vi "querySignalInterface.vi"(8 "error in (no error)":errorcluster, 11 "IBaseObject in":refnum<class "IBaseObject.lvclass">) -> (0 "error out":errorcluster, 2 "ISignal out":refnum<class "ISignal.lvclass">, 3 "IBaseObject out":refnum<class "IBaseObject.lvclass">)   [LabVIEW 2022 SP3, in "openDAQ.lvlib" / "IBaseObject.lvlib" / "IBaseObject.lvclass"]
uses:
  <instrlib>/openDAQ/Public/Classes/IBaseObject/IBaseObject.lvclass
  <instrlib>/openDAQ/Public/Classes/IBaseObject/IBaseObject.lvclass/IBaseObject.ctl
  <instrlib>/openDAQ/Binaries/Windows/x86/copendaq32.dll
  <instrlib>/openDAQ/Public/Classes/ISignal/ISignal.lvclass
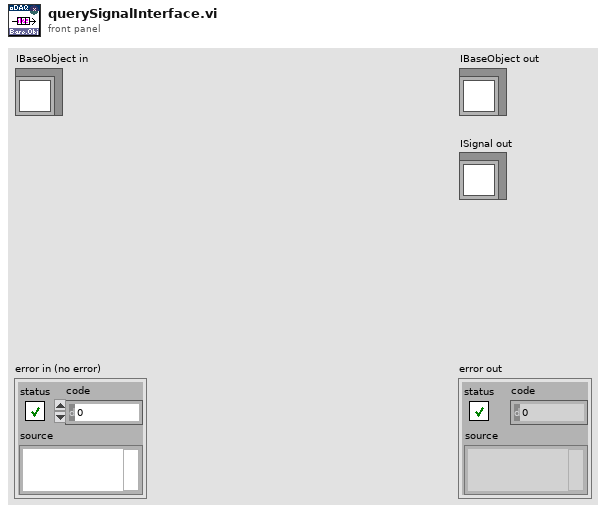
[diagram p1: front panel]
types:
  T1 = enum16{"big-endian, network order", "native, host order", "little-endian"}
  T2 = cluster{"status":bool, "code":u32, "source":string}
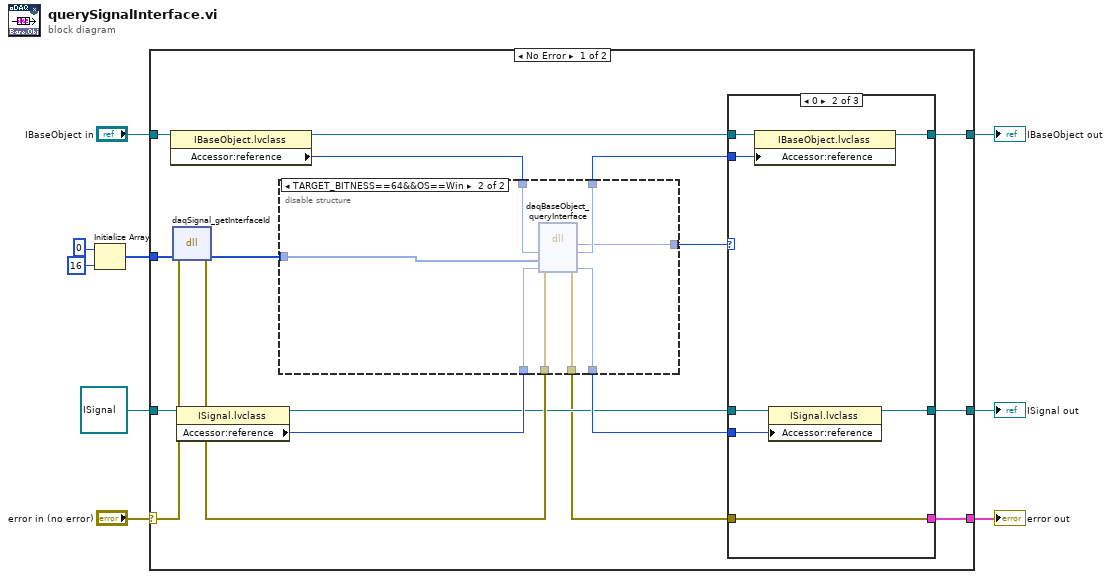
[diagram p0: block diagram]
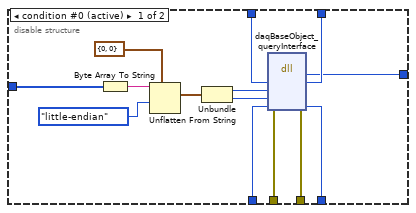
[diagram p2: hidden frame]
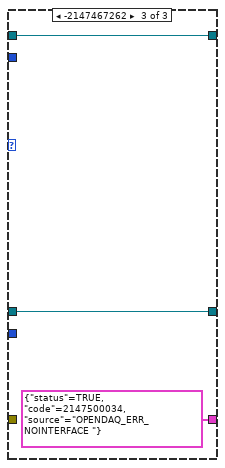
[diagram p4: hidden frame]
diagram:
  n1 = Initialize Array(u8 0, 16 ("dimension size")) -> (w1:u8[])
  n2 = case shown="No Error" "error in (no error)" {
    selector: "error in (no error)" -> [w22 w64]
    tunnel: [w12 w64] -> w8
    tunnel: [w19 w63] -> w6
    tunnel: "IBaseObject in" -> [w26 w63]
    tunnel: refnum<class "ISignal.lvclass"> refnum ("openDAQ.lvlib:IBaseObject.lvlib:IPropertyObject.lvlib:IComponent.lvlib:ISignal.lvlib:ISignal.lvclass") -> [w25 w62]
    tunnel: [w15 w62] -> w4
    tunnel: w1 -> [w11 _]
    frame No Error {
      n3 = property class="IBaseObject.lvclass"(reference=w26) -> (reference out=w20:refnum<class "IBaseObject.lvclass">, "Accessor:reference"=w24:i64)  [unwired: 1 in, 1 out]
      n4 = dll-call lib="C:/Program Files (x86)/National Instruments/LabVIEW 2022/instr.lib/openDAQ/Binaries/Windows/x86/copendaq*.*" fn="daqSignal_getInterfaceId"(error in=w22, "id"=w11) -> (error out=w21:errorcluster, "id"=w10:u8[])  [unwired: 3 in, 1 out]
      n5 = property class="ISignal.lvclass"(reference=w25) -> (reference out=w16:refnum<class "ISignal.lvclass">, "Accessor:reference"=w23:i64)  [unwired: 1 in, 1 out]
      n6 = disable-structure shown="TARGET_BITNESS==64&&OS==Win" {
        disable-tunnel: w24 -> [w40 w46]
        disable-tunnel: w23 -> [w39 w43]
        disable-tunnel: w21 -> [w38 w48]
        disable-tunnel: [w37 w45] -> w18
        disable-tunnel: [w36 w42] -> w17
        disable-tunnel: [w35 w44] -> w14
        disable-tunnel: [w34 w47] -> w13
        disable-tunnel: w10 -> [w30 w41]
        frame condition #0 (active) {
          n7 = Byte Array To String(unsigned byte array=w30) -> (string=w33:string)
          n8 = Unflatten From String(type=cluster{u64, u64} {0, 0}, binary string=w33, byte order (0:big-endian, network order)=T1."little-endian") -> (value=w31:cluster{u64, u64})  [unwired: 2 in, 2 out]
          n9 = Unbundle(w31) -> (w29:u64, w28:u64)
          n10 = dll-call lib="C:/Program Files (x86)/National Instruments/LabVIEW 2022/instr.lib/openDAQ/Binaries/Windows/x86/copendaq*.*" fn="daqBaseObject_queryInterface"(error in=w38, "self"=w40, "intfId1"=w29, "intfId2"=w28, "interfacePtr"=w39) -> (error out=w34:errorcluster, "return type"=w35:u32, "self"=w37:i64, "interfacePtr"=w36:i64)  [unwired: 4 in, 1 out]
        }
        frame condition #1 {
          n11 = dll-call lib="C:/Program Files (x86)/National Instruments/LabVIEW 2022/instr.lib/openDAQ/Binaries/Windows/x86/copendaq*.*" fn="daqBaseObject_queryInterface"(error in=w48, "self"=w46, "intfId"=w41, "interfacePtr"=w43) -> (error out=w47:errorcluster, "return type"=w44:u32, "self"=w45:i64, "interfacePtr"=w42:i64)  [unwired: 3 in, 1 out]
        }
      }
      n12 = case shown="0" w14 {
        tunnel: w20 -> [w50 w58 w61]
        tunnel: [w50 w57 w61] -> w19
        tunnel: w18 -> [_ w56 _]
        tunnel: w17 -> [_ w55 _]
        tunnel: w16 -> [w49 w54 w60]
        tunnel: [w49 w53 w60] -> w15
        tunnel: w13 -> [w51 w52 _]
        tunnel: [w51 w52 T2 {"status"=TRUE, "code"=2147500034, "source"="OPENDAQ_ERR_NOINTERFACE "} ("error out")] -> w12
        frame Default {
        }
        frame 0 {
          n13 = property class="IBaseObject.lvclass"(reference=w58, "Accessor:reference"=w56) -> (reference out=w57:refnum<class "IBaseObject.lvclass">)  [unwired: 1 in, 1 out]
          n14 = property class="ISignal.lvclass"(reference=w54, "Accessor:reference"=w55) -> (reference out=w53:refnum<class "ISignal.lvclass">)  [unwired: 1 in, 1 out]
        }
        frame -2147467262 {
        }
      }
    }
    frame Error {
    }
  }
  "error out" <- w8
  "IBaseObject out" <- w6
  "ISignal out" <- w4
